vi "update config.vi"(8 "error in (no error)":errorcluster, 10 "user configurations":T2={"vst_device"=["VST_1", "VST_2"], "RF gain "=10.0, "buffer size"=524288, "center frequency (Hz) "=1000000000.0, "P2P sample rate"=200000000.0, "mode"=enum."5785 - 2*180MHz", "devicess"=["IF_transiver_0", "IF_transiver_1", "IF_transiver_2"], "file paths"=[path "C:/Users/PXIe8108_Demo/Documents/CHAIM DATA/chaim/5785_sync_for_elbit/data/pdw_test_file.tdms", path "C:/Users/PXIe8108_Demo/Documents/CHAIM DATA/chaim/5785_sync_for_elbit/data/pdw_test_file_1.tdms", path "C:/Users/PXIe8108_Demo/Documents/CHAIM DATA/chaim/5785_sync_for_elbit/data/pdw_test_file_2.tdms", path "C:/Users/PXIe8108_Demo/Documents/CHAIM DATA/chaim/5785_sync_for_elbit/data/pdw_test_file_3.tdms", path "C:/Users/PXIe8108_Demo/Documents/CHAIM DATA/chaim/5785_sync_for_elbit/data/pdw_test_file_4.tdms"], "gen for df"=FALSE}, 11 "5785_3.2GHz_one channel in":refnum<class "5785_3.2GHz_one channel.lvclass">) -> (0 "error out":errorcluster, 1 "min frequency":dbl, 2 "max frequency":dbl, 3 "5785_3.2GHz_one channel out":refnum<class "5785_3.2GHz_one channel.lvclass">)   [LabVIEW 2021, in "5785_3.2GHz_one channel.lvclass"]
uses:
  5785_3.2GHz_one channel.lvclass
  <vilib>/userdefined/High Color/nirio_resource_hc.ctl
  5785_3.2GHz_one channel.lvclass/5785_3.2GHz_one channel.ctl
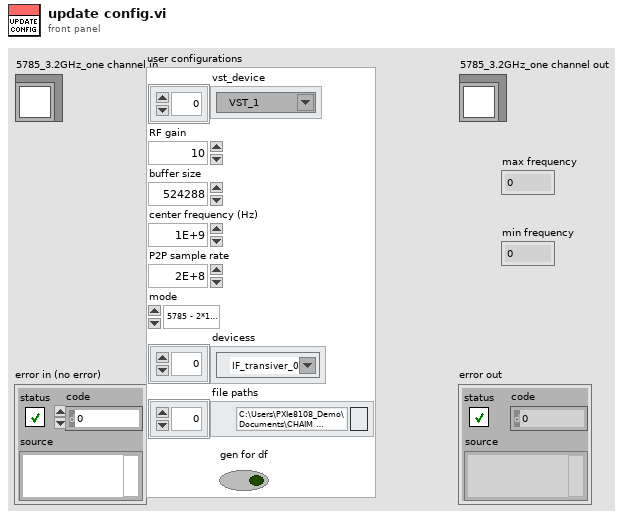
[diagram p1: front panel]
types:
  T1 = typedef "nirio_resource_hc.ctl" = tag
  T2 = cluster{"vst_device":refnum<k15>[], "RF gain ":dbl, "buffer size":u32, "center frequency (Hz) ":dbl, "P2P sample rate":dbl, "mode":enum16{"USRP - 180MHz", "5785 - 2*180MHz", "5785 - 3.2GHz", "P2P - VST"}, "devicess":T1[], "file paths":path[], "gen for df":bool}
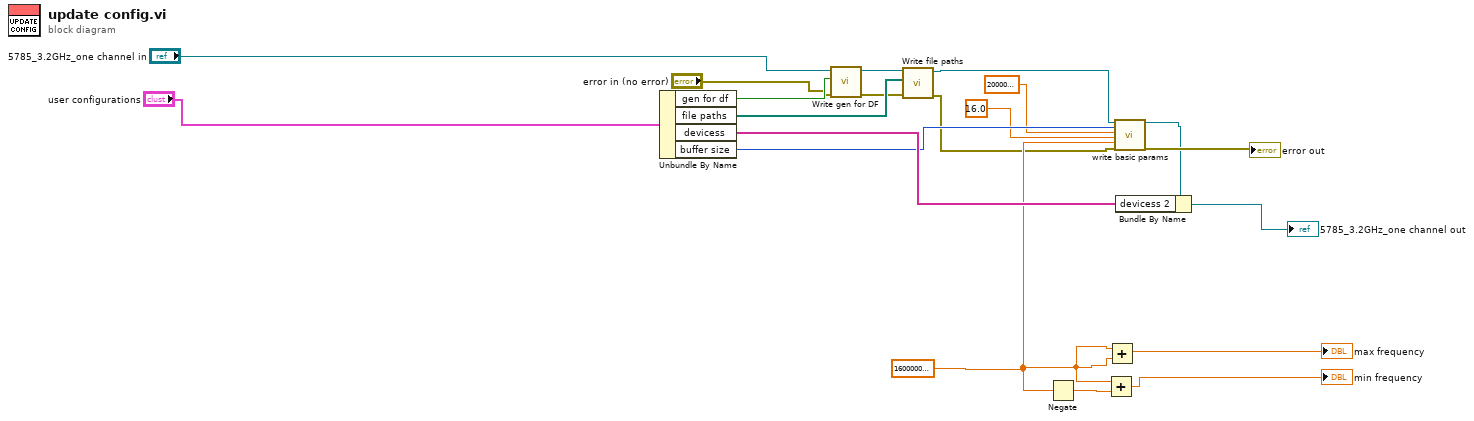
[diagram p0: block diagram]
diagram:
  w11 = 1600000000.0
  n1 = Unbundle By Name("user configurations") -> ("gen for df"=w4:bool, "file paths"=w8:path[], "devicess"=w20:T1[], "buffer size"=w14:u32)
  n2 = call-dynamic "Write gen for DF.vi"("error in (no error)"="error in (no error)", "gen for DF"=w4, "device_type in"="5785_3.2GHz_one channel in") -> ("error out"=w3:errorcluster, "device_type out"=w6:refnum<class "5785_3.2GHz_one channel.lvclass">)  [unwired: 7 in]
  n3 = call-dynamic "Write file paths.vi"("error in (no error)"=w3, "file paths"=w8, "device_type in"=w6) -> ("error out"=w2:errorcluster, "device_type out"=w7:refnum<class "5785_3.2GHz_one channel.lvclass">)  [unwired: 7 in]
  n4 = Negate(x=w11) -> (-x=w19:dbl)
  n5 = Add(x=w11, y=w19) -> (x+y=→"min frequency":dbl)
  n6 = Add(x=w11, y=w11) -> (x+y=→"max frequency":dbl)
  n7 = call-dynamic "write basic params.vi"("device_type in"=w7, "buffer size"=w14, "Fs  FPGA"=200000000.0, "SPC"=16.0 ("Fs  FPGA"), "center frequency (Hz)"=w11, "error in (no error)"=w2) -> ("device_type out"=w9:refnum<class "5785_3.2GHz_one channel.lvclass">, "error out"=→"error out":errorcluster)  [unwired: 12 in]
  n8 = Bundle By Name(cluster=w9, "devicess 2"=w20) -> (→"5785_3.2GHz_one channel out":refnum<class "5785_3.2GHz_one channel.lvclass">)
